vi "dR_R_for_ThemalImaging(u8).vi"(10 "DR/R parameter":T2, 11 "数据值引用":refnum<data-value>) -> (3 "Image Dst Out":T1)   [LabVIEW 2011]
uses:
  <vilib>/vision/Image Controls.llb/IMAQ Image.ctl
  <vilib>/vision/NI_Vision_Development_Module.lvlib
panel:
  out "数组 2":bool[](array[boolean])
  out "Image":T1(plugin-control)
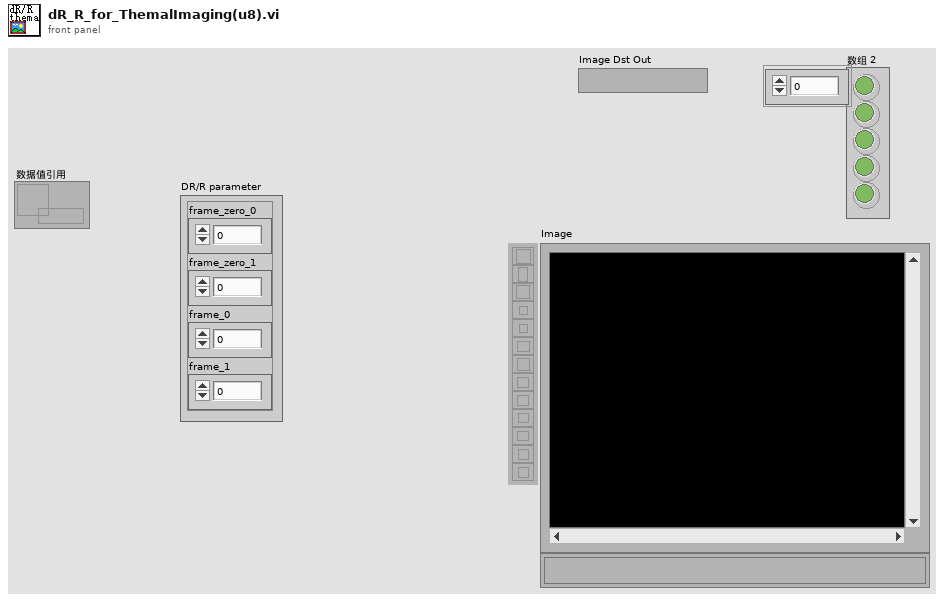
[diagram p1: front panel]
types:
  T1 = typedef "IMAQ Image.ctl" = refnum<image>
  T2 = cluster{"frame_zero_0":i32, "frame_zero_1":i32, "frame_0":i32, "frame_1":i32}
  T3 = typedef "Image Type" = u32
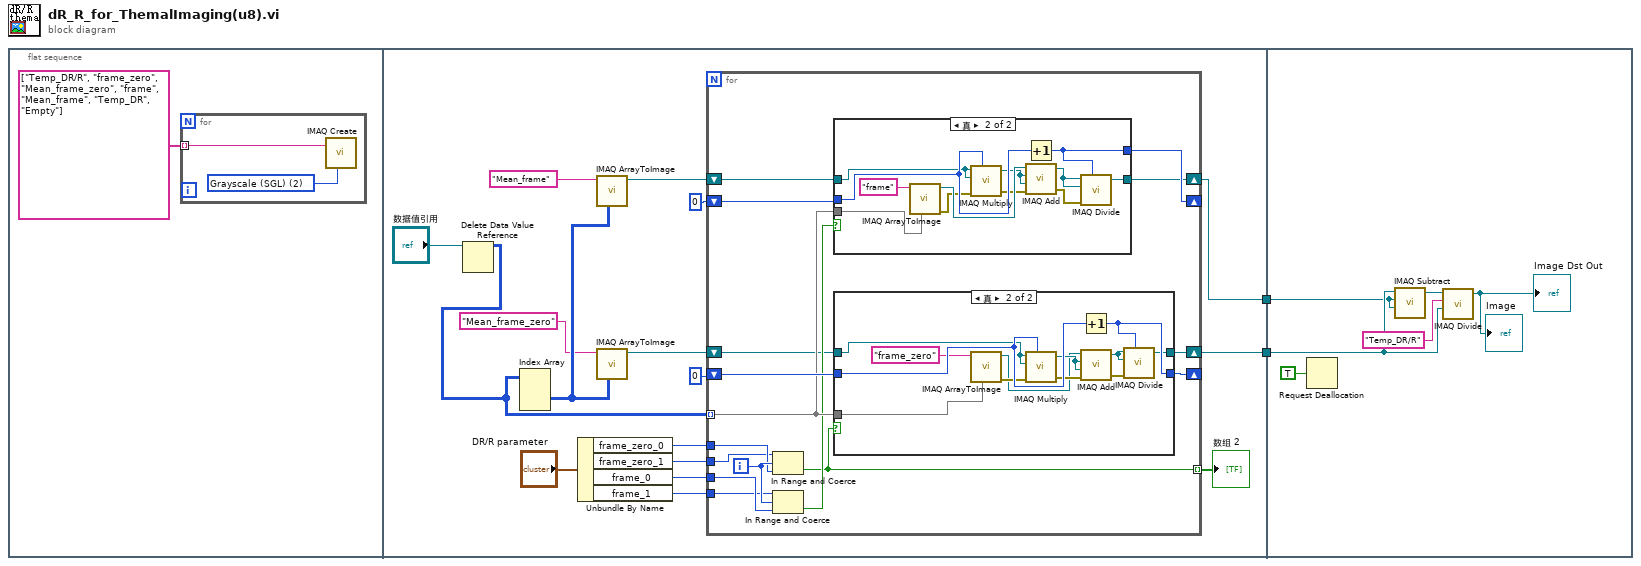
[diagram p0: block diagram]
diagram:
  n1 = flat-sequence {
    tunnel: [w14] -> w2
    tunnel: [w8] -> w1
    tunnel: w2 -> [w68]
    tunnel: w1 -> [w67]
    frame #0 {
      n2 = for {
        tunnel: string[] ["Temp_DR/R", "frame_zero", "Mean_frame_zero", "frame", "Mean_frame", "Temp_DR", "Empty"] ("添加的数组") -> [w4] mode=indexing
        w5 = T3 2 items=["Grayscale (U8)", "Grayscale (I16)", "Grayscale (SGL)", "Complex (CSG)", "RGB (U32)", "HSL (U32)", "RGB (U64)", "Grayscale (U16)"] ("Image Type")
        n3 = call "IMAQ Create"("Image Name"=w4, "Image Type"=w5) -> ()  [unwired: 3 in, 2 out]
      }
    }
    frame #1 {
      n4 = Delete Data Value Reference(data value reference="数据值引用") -> (data value=w6:u8[][][])  [unwired: 1 in, 1 out]
      n5 = Index Array(array=w6) -> (element=w13:u8[][])  [unwired: 3 in]
      n6 = Unbundle By Name("DR/R parameter") -> ("frame_zero_0"=w21:i32, "frame_zero_1"=w20:i32, "frame_0"=w18:i32, "frame_1"=w17:i32)
      n7 = call "IMAQ ArrayToImage"("Image Pixels (Float)"=w13, "Image"="Mean_frame" ("Image Name")) -> ("Image Out"=w10:T1)  [unwired: 8 in, 1 out]
      n8 = call "IMAQ ArrayToImage"("Image Pixels (Float)"=w13, "Image"="Mean_frame_zero" ("Image Name")) -> ("Image Out"=w9:T1)  [unwired: 8 in, 1 out]
      n9 = for {
        tunnel: w6 -> [w35] mode=indexing
        tunnel: w21 -> [w30]
        tunnel: w20 -> [w29]
        shift-right: [w37] -> _
        shift-left: 0 -> [w38]
        tunnel: w18 -> [w28]
        tunnel: w17 -> [w27]
        shift-right: [w33] -> _
        shift-left: 0 -> [w34]
        tunnel: [w31] -> w15 mode=indexing
        shift-right: [w26] -> w14
        shift-left: w9 -> [w25]
        shift-right: [w24] -> w8
        shift-left: w10 -> [w23]
        i -> [w36]
        n10 = In Range and Coerce(upper limit=w29, x=w36, lower limit=w30) -> (In Range?=w31:bool)  [unwired: 1 out]
        n11 = In Range and Coerce(upper limit=w27, x=w36, lower limit=w28) -> (In Range?=w32:bool)  [unwired: 1 out]
        n12 = case shown="真" w32 {
          tunnel: w35 -> [_ w52]
          tunnel: w34 -> [w40 w50]
          tunnel: [w40 w44] -> w33
          tunnel: [w39 w42] -> w24
          tunnel: w23 -> [w39 w41]
          frame False {
          }
          frame True {
            n13 = call "IMAQ ArrayToImage"("Image Pixels (Float)"=w52, "Image"="frame" ("Image Name")) -> ("error out"=w45:errorcluster, "Image Out"=w49:T1)  [unwired: 8 in]
            n14 = call "IMAQ Multiply"("Image Src A"=w41, "Constant"=w50, "Image Dst"=w41, "error in (no error)"=w45) -> ("Image Dst Out"=w48:T1, "error out"=w46:errorcluster)  [unwired: 3 in]
            n15 = Increment(x=w50) -> (x+1=w44:i32)
            n16 = call "IMAQ Add"("Image Src A"=w49, "Image Dst"=w48, "Image Src B"=w48, "error in (no error)"=w46) -> ("Image Dst Out"=w43:T1, "error out"=w47:errorcluster)  [unwired: 3 in]
            n17 = call "IMAQ Divide"("Image Src A"=w43, "Constant"=w44, "Image Dst"=w43, "error in (no error)"=w47) -> ("Image Dst Out"=w42:T1)  [unwired: 3 in, 1 out]
          }
        }
        n18 = case shown="真" w31 {
          tunnel: w35 -> [_ w66]
          tunnel: w38 -> [w54 w65]
          tunnel: [w54 w61] -> w37
          tunnel: [w53 w56] -> w26
          tunnel: w25 -> [w53 w55]
          frame False {
          }
          frame True {
            n19 = call "IMAQ ArrayToImage"("Image Pixels (Float)"=w66, "Image"="frame_zero" ("Image Name")) -> ("error out"=w62:errorcluster, "Image Out"=w57:T1)  [unwired: 8 in]
            n20 = call "IMAQ Multiply"("Image Src A"=w55, "Constant"=w65, "Image Dst"=w55, "error in (no error)"=w62) -> ("Image Dst Out"=w58:T1, "error out"=w63:errorcluster)  [unwired: 3 in]
            n21 = Increment(x=w65) -> (x+1=w61:i32)
            n22 = call "IMAQ Add"("Image Src A"=w57, "Image Dst"=w58, "Image Src B"=w58, "error in (no error)"=w63) -> ("Image Dst Out"=w59:T1, "error out"=w64:errorcluster)  [unwired: 3 in]
            n23 = call "IMAQ Divide"("Image Src A"=w59, "Constant"=w61, "Image Dst"=w59, "error in (no error)"=w64) -> ("Image Dst Out"=w56:T1)  [unwired: 3 in, 1 out]
          }
        }
      }
      "数组 2" <- w15
    }
    frame #2 {
      n24 = Request Deallocation(TRUE ("标志")) -> ()
      n25 = call "IMAQ Subtract"("Image Src A"=w68, "Image Dst"=w67, "Image Src B"=w67) -> ("Image Dst Out"=w72:T1)  [unwired: 4 in, 1 out]
      n26 = call "IMAQ Divide"("Image Src A"=w72, "Image Dst"="Temp_DR/R" ("Image Name"), "Image Src B"=w68) -> ("Image Dst Out"=→"Image Dst Out" →"Image":T1)  [unwired: 4 in, 1 out]
    }
  }
